vi "tio32_GetBoardCount.vi"(8 "error in (no error)":errorcluster, 11 "VISA resource name":refnum<visa-resource-name>) -> (0 "error out":errorcluster, 1 "# of boards":i32, 2 "return":i32=666, 3 "VISA resource name out":refnum<visa-resource-name>, 4 "Address":i32[](array[numeric]) format="%x")   [LabVIEW 2011]
doc: "DLL tio32.DLL\nFunction INT16TYPE WINAPI tio32_GetBoardCount(INT16TYPE *pNumberOfBoards);\n\nGet the number of connected TI DAQ-boards."
uses:
  l_pse_dll/Tio32.dll
panel:
  # "tio32_GetBoardCount"
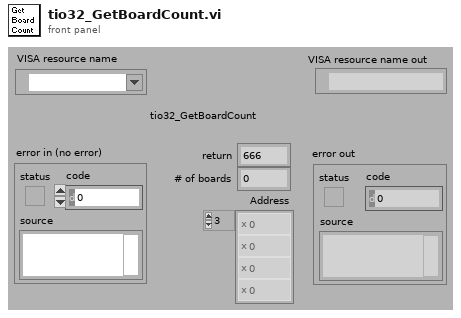
[diagram p1: front panel]
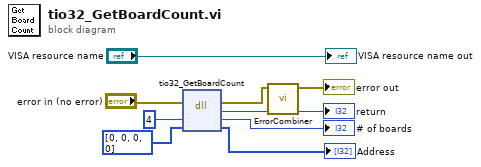
[diagram p0: block diagram]
diagram:
  n1 = dll-call lib="C:/Users/Ikaika's/Documents/DCC/Apps/INA231/INA231-SFT-rev1/INA231-Sourcecode-rev1/INA231/Shell Resources/l_pse_dll/Tio32.dll" fn="tio32_GetBoardCount"(error in="error in (no error)", "pCount"=i16 4, "pAddr"=i32[] [0, 0, 0, 0]) -> (error out=w4:errorcluster, "Rückgabetyp"=w5:i32, "pCount"=→"# of boards":i32, "pAddr"=→"Address":i32[])  [unwired: 2 in, 1 out]
  n2 = call "ErrorCombiner.vi"("Return In"=w5, "error in (no error)"=w4) -> ("Return Out"=→"return":i32, "error out"=→"error out":errorcluster)  [unwired: 8 in]
  "VISA resource name out" <- "VISA resource name"
